vi "Render Picture.vi"(11 "Circle In":refnum<class "Circle.lvclass">) -> (1 "Picture":picture, 3 "Circle Out":refnum<class "Circle.lvclass">)   [LabVIEW 2017, in "Circle.lvclass"]
doc: "This VI is analogous to a pure virtual function. It does no real work and exists only to be overridden by its descendant classes."
uses:
  Circle.lvclass
  Circle.lvclass/Circle.ctl
  Point/Point.lvclass
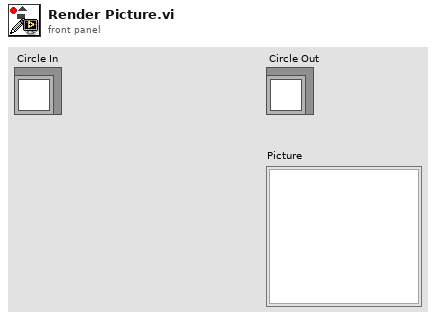
[diagram p1: front panel]
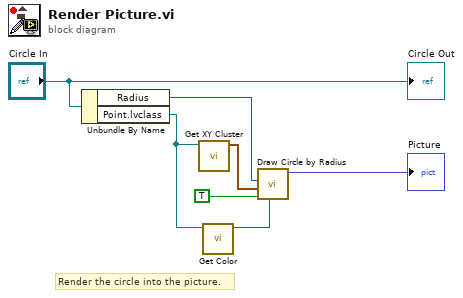
[diagram p0: block diagram]
diagram:
  # "Render the circle into the picture."
  n1 = Unbundle By Name("Circle In") -> ("Radius"=w5:u16, "Point.lvclass"=w2:refnum<class "Point.lvclass">)
  n2 = call "Get XY Cluster.vi"("Point.lvclass"=w2) -> ("XY Cluster"=w6:cluster{"X":i16, "Y":i16})  [unwired: 10 in]
  n3 = call "Get Color.vi"("Point"=w2) -> ("Color"=w1:u32)  [unwired: 10 in]
  n4 = call <vilib>:"Draw Circle by Radius.vi"("color(black)"=w1, "fill?(F)"=TRUE, "pixel center"=w6, "radius"=w5) -> ("new picture"=→"Picture":picture)  [unwired: 4 in, 3 out]
  "Circle Out" <- "Circle In"
